vi "Get Device Name.vi"(8 "error in (no error)":errorcluster caption="错误输入（无错误）", 11 "Screen 输入":refnum<class "Screen.lvclass"> caption="DNL_LabVIEW Object in") -> (0 "error out":errorcluster caption="错误输出", 2 "DeviceName":string, 3 "Screen 输出":refnum<class "Screen.lvclass"> caption="DNL_LabVIEW Object out")   [LabVIEW 2011, in "Screen.lvclass"]
uses:
  Screen.lvclass
  Screen.lvclass/Screen.ctl
  System.Windows.Forms
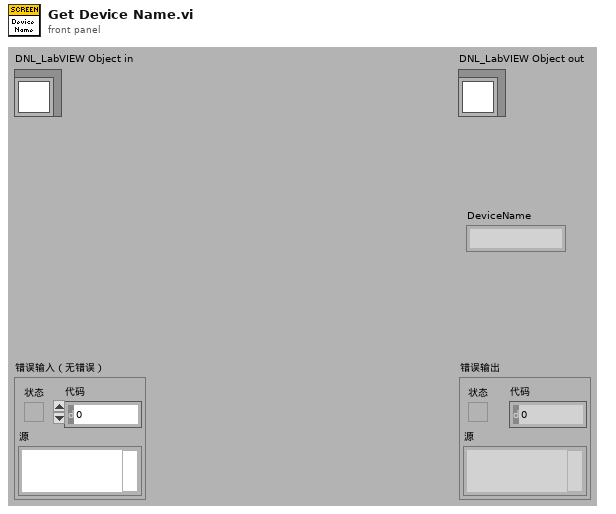
[diagram p1: front panel]
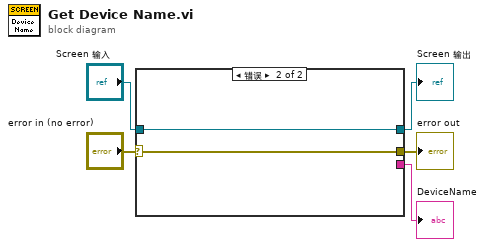
[diagram p0: block diagram]
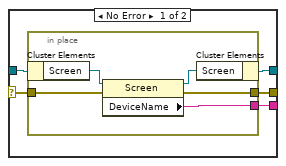
[diagram p2: hidden frame]
diagram:
  n1 = case shown="错误" "error in (no error)" {
    selector: "error in (no error)" -> [w7 w17]
    tunnel: [w6 w17] -> w4
    tunnel: [w8 w16] -> w2
    tunnel: "Screen 输入" -> [w10 w16]
    tunnel: [w9 _] -> w1
    frame No Error {
      n2 = in-place {
        in-place-border: [w13] -> w9
        in-place-border: w7 -> [w12]
        in-place-border: [w11] -> w6
        n3 = in-place-cluster #1(w10) -> ("Screen"=w15:refnum<k24>)
        n4 = property class="Screen"(reference=w15, error in=w12) -> (reference out=w14:refnum<k24>, error out=w11:errorcluster, "DeviceName"=w13:string)
        n5 = in-place-cluster #1("Screen"=w14) -> (w8:refnum<class "Screen.lvclass">)
      }
    }
    frame Error {
    }
  }
  "error out" <- w4
  "Screen 输出" <- w2
  "DeviceName" <- w1
